vi "absolute value con deadband.vi"(11 "Joystick Value":dbl) -> (3 "Val":dbl)   [LabVIEW 2019]
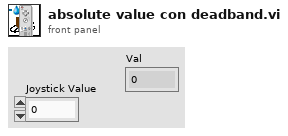
[diagram p1: front panel]
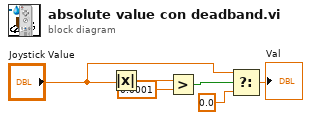
[diagram p0: block diagram]
diagram:
  n1 = Absolute Value(x="Joystick Value") -> (abs(x)=w2:dbl)
  n2 = Greater?(x=w2, y=0.0001) -> (0:w4:bool)
  n3 = Select(t="Joystick Value", s=w4, f=0.0) -> (s? t:f=→"Val":dbl)
